vi "Gate delay Position.vi"(8 "error in (no error)":errorcluster, 10 "i (0)":T1, 11 "VISA resource name":refnum<visa-resource-name>) -> (0 "error out":errorcluster, 2 "output":dbl, 3 "VISA resource name out":refnum<visa-resource-name>)   [LabVIEW 2015, in "SR400.lvlib"]
doc: "The GZ command returns the gate delay position\nduring a scan. i = 0 or 1 designates A gate or B\ngate and is required. If gate i is in the SCAN\nmode, its current delay position during a scan is\nread. If the counters are in reset or the gate is not\nin the SCAN mode, the GZ command returns the\nstarting delay position (same as GD command).\nThe GZ command is a read only command."
uses:
  SR400.lvlib
  Typedefs/Gate.ctl
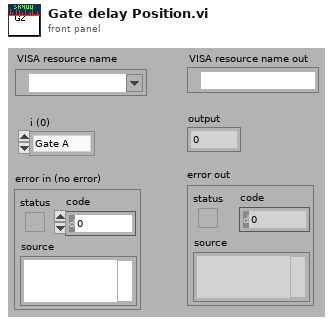
[diagram p1: front panel]
types:
  T1 = typedef "SR400.lvlib/Gate.ctl" = enum16{"Gate A", "Gate B"}
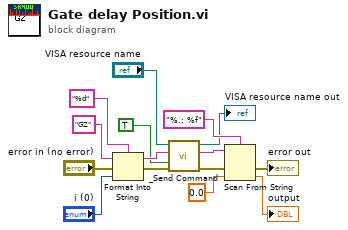
[diagram p0: block diagram]
diagram:
  n1 = Format Into String(format string="%d", initial string="GZ" ("command"), error in="error in (no error)", "i (0)") -> (resulting string=w6:string, error out=w5:errorcluster)
  n2 = call "_Send Command.vi"("error in (no error)"=w5, "Query? (F)"=TRUE, "Command"=w6, "VISA resource name"="VISA resource name") -> ("error out"=w2:errorcluster, "Response"=w3:string, "VISA resource name out"=→"VISA resource name out":refnum<visa-resource-name>)  [unwired: 5 out]
  n3 = Scan From String(format string="%.; %f", input string=w3, error in=w2, default 1=0.0 ("default value 1")) -> (error out=→"error out":errorcluster, output 1=→"output":dbl)  [unwired: 1 in, 2 out]
